vi "ADCP_CM_Packet_To_Processed_Bytes.vi"(8 "error in (no error)":errorcluster, 10 "Connection Management":T1, 11 "ADCP in":refnum<class "ADCP.lvclass">) -> (0 "error out":errorcluster, 2 "Processed Packet":u8[](array[numeric]), 3 "ADCP out":refnum<class "ADCP.lvclass">)   [LabVIEW 2017, in "ADCP.lvclass"]
uses:
  ADCP.lvclass
  ADCP.lvclass/ADCP.ctl
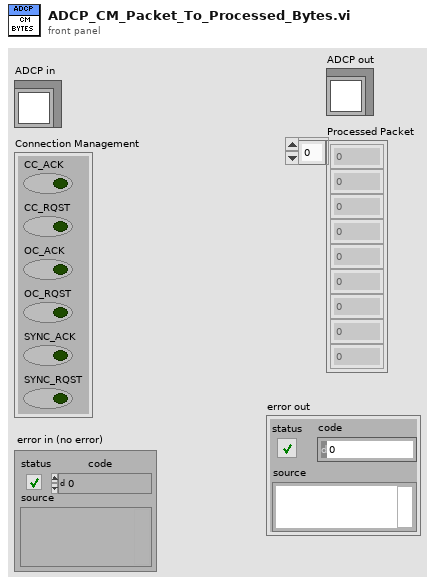
[diagram p1: front panel]
types:
  T1 = cluster{"CC_ACK":bool, "CC_RQST":bool, "OC_ACK":bool, "OC_RQST":bool, "SYNC_ACK":bool, "SYNC_RQST":bool}
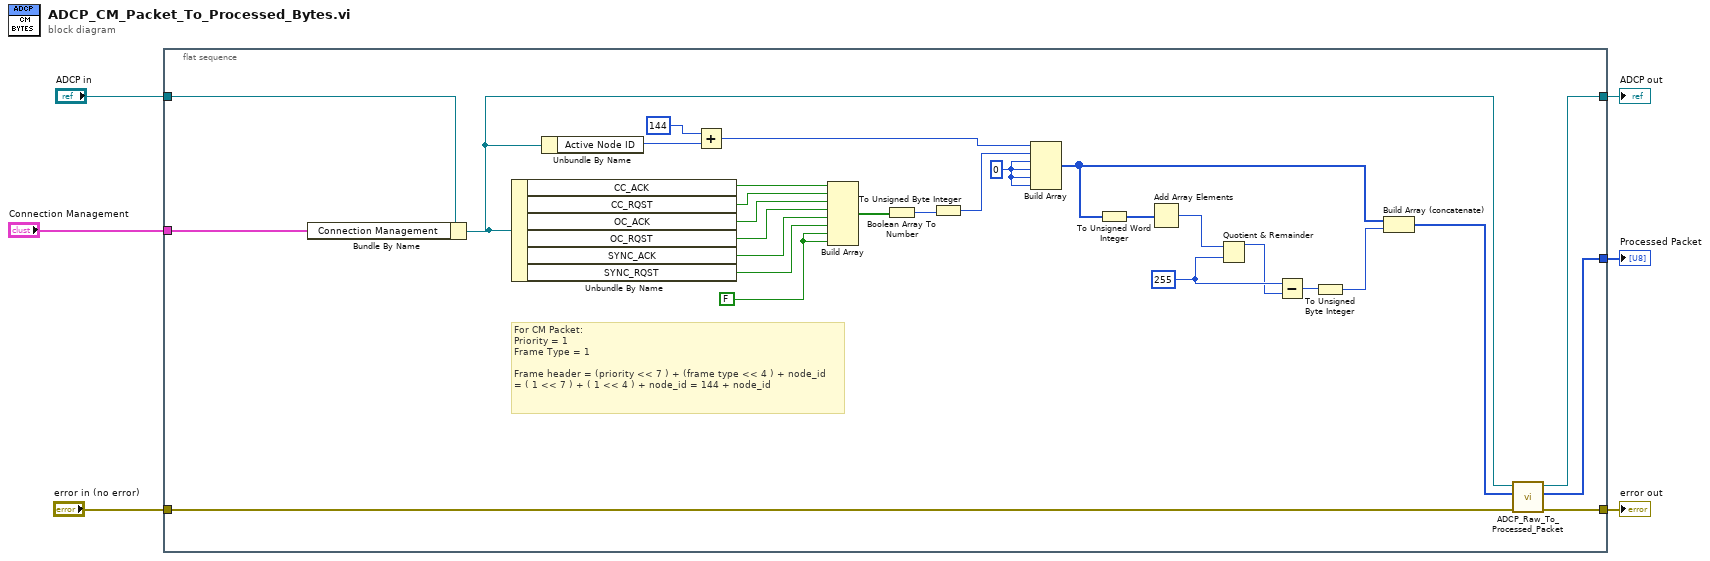
[diagram p0: block diagram]
diagram:
  n1 = flat-sequence {
    tunnel: "ADCP in" -> [w12]
    tunnel: "error in (no error)" -> [w17]
    tunnel: [w16] -> w3
    tunnel: [w15] -> w4
    tunnel: [w13] -> w2
    tunnel: "Connection Management" -> [w10]
    frame #0 {
      w22 = u16 255 ("y")
      w25 = u8 0 ("element")
      w29 = FALSE
      # "For CM Packet:\nPriority = 1\nFrame Type = 1\n\nFrame header = (priority << 7 ) + (frame type << 4 ) + node_id\n= ( 1 << 7 ) + ( 1 << 4 ) + node_id = 144 + node_id"
      n2 = Bundle By Name(cluster=w12, "Connection Management"=w10) -> (w11:refnum<class "ADCP.lvclass">)
      n3 = Unbundle By Name(w11) -> ("CC_ACK"=w35:bool, "CC_RQST"=w34:bool, "OC_ACK"=w33:bool, "OC_RQST"=w32:bool, "SYNC_ACK"=w31:bool, "SYNC_RQST"=w30:bool)
      n4 = Unbundle By Name(w11) -> ("Active Node ID"=w9:u8)
      n5 = Add(x=u8 144, y=w9) -> (x+y=w8:u8)
      n6 = Build Array(w35, w34, w33, w32, w31, w30, w29, w29) -> (w28:bool[])
      n7 = Boolean Array To Number(Boolean array=w28) -> (number=w27:u32)
      n8 = To Unsigned Byte Integer(number=w27) -> (unsigned 8bit integer=w26:u8)
      n9 = Build Array(w8, w26, w25, w25, w25, w25) -> (w20:u8[])
      n10 = To Unsigned Word Integer(number=w20) -> (unsigned 16bit integer=w24:u16[])
      n11 = Add Array Elements(numeric array=w24) -> (sum=w23:u16)
      n12 = Quotient & Remainder(x=w23, y=w22) -> (x-y*floor(x/y)=w21:u16)  [unwired: 1 out]
      n13 = Subtract(x=w22, y=w21) -> (x-y=w19:u16)
      n14 = To Unsigned Byte Integer(number=w19) -> (unsigned 8bit integer=w18:u8)
      n15 = Build Array (concatenate)(w20, w18) -> (w14:u8[])
      n16 = call "ADCP_Raw_To_Processed_Packet.vi"("error in (no error)"=w17, "Raw Packet"=w14, "ADCP in"=w11) -> ("error out"=w16:errorcluster, "Processed Packet"=w13:u8[], "ADCP out"=w15:refnum<class "ADCP.lvclass">)  [unwired: 6 in]
    }
  }
  "ADCP out" <- w4
  "error out" <- w3
  "Processed Packet" <- w2
